vi "主动发送数据生成Condition(子VI).vi"(8 "数据发送协议":enum16{"2005-212协议", "2017-212协议"}(ring)=enum."2017-212协议", 9 "database":string, 10 "Label.Text":string, 11 "数值":i32) -> (3 "CONDITION":string)   [LabVIEW 2016, in "数据传输系统.lvlib"]
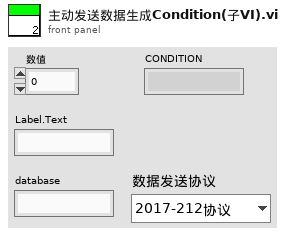
[diagram p1: front panel]
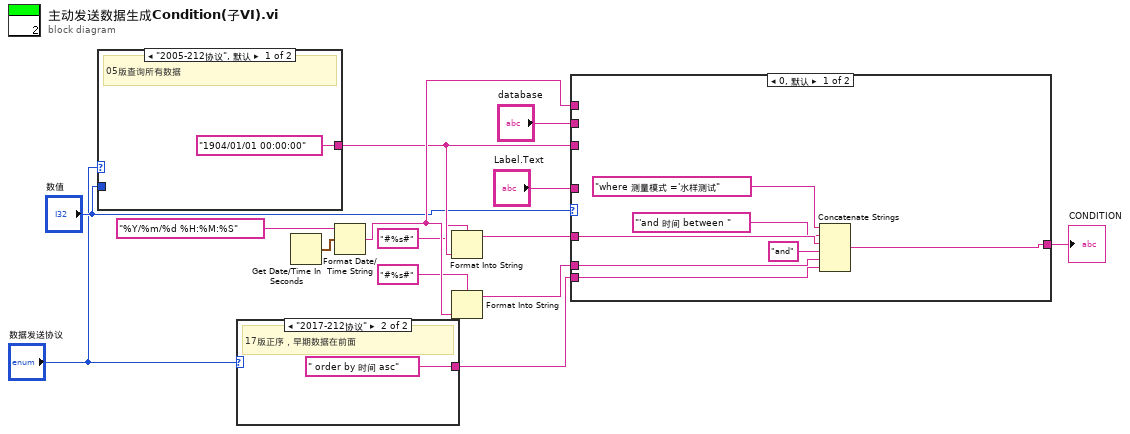
[diagram p0: block diagram]
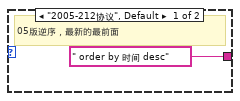
[diagram p2: hidden frame]
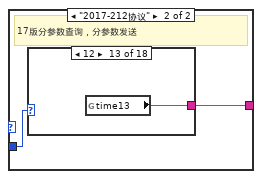
[diagram p3: hidden frame]
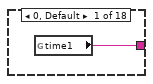
[diagram p4: hidden frame]
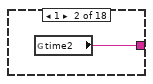
[diagram p5: hidden frame]
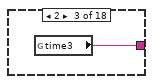
[diagram p6: hidden frame]
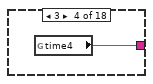
[diagram p7: hidden frame]
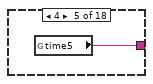
[diagram p8: hidden frame]
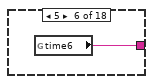
[diagram p9: hidden frame]
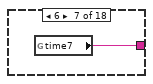
[diagram p10: hidden frame]
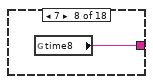
[diagram p11: hidden frame]
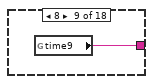
[diagram p12: hidden frame]
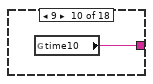
[diagram p13: hidden frame]
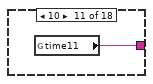
[diagram p14: hidden frame]
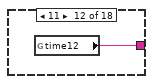
[diagram p15: hidden frame]
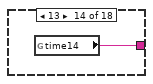
[diagram p16: hidden frame]
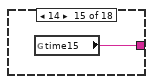
[diagram p17: hidden frame]
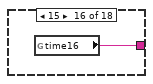
[diagram p18: hidden frame]
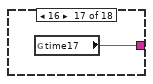
[diagram p19: hidden frame]
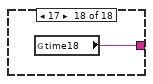
[diagram p20: hidden frame]
diagram:
  n1 = case shown="\"2005-212协议\", 默认" "数据发送协议" {
    tunnel: ["1904/01/01 00:00:00" w17] -> w13
    tunnel: "数值" -> [_ w16]
    frame "2005-212协议", Default {
      # "05版查询所有数据"
    }
    frame "2017-212协议" {
      # "17版分参数查询，分参数发送"
      n2 = case shown="12" w16 {
        tunnel: [w18 w19 w20 w21 w22 w23 w24 w25 w26 w27 w28 w29 w30 w31 w32 w33 w34 w35] -> w17
        frame 0, Default {
          n3 = global read "全局 水样时间.vi" "time1"() -> (w18:string)
        }
        frame 1 {
          n4 = global read "全局 水样时间.vi" "time2"() -> (w19:string)
        }
        frame 2 {
          n5 = global read "全局 水样时间.vi" "time3"() -> (w20:string)
        }
        frame 3 {
          n6 = global read "全局 水样时间.vi" "time4"() -> (w21:string)
        }
        frame 4 {
          n7 = global read "全局 水样时间.vi" "time5"() -> (w22:string)
        }
        frame 5 {
          n8 = global read "全局 水样时间.vi" "time6"() -> (w23:string)
        }
        frame 6 {
          n9 = global read "全局 水样时间.vi" "time7"() -> (w24:string)
        }
        frame 7 {
          n10 = global read "全局 水样时间.vi" "time8"() -> (w25:string)
        }
        frame 8 {
          n11 = global read "全局 水样时间.vi" "time9"() -> (w26:string)
        }
        frame 9 {
          n12 = global read "全局 水样时间.vi" "time10"() -> (w27:string)
        }
        frame 10 {
          n13 = global read "全局 水样时间.vi" "time11"() -> (w28:string)
        }
        frame 11 {
          n14 = global read "全局 水样时间.vi" "time12"() -> (w29:string)
        }
        frame 12 {
          n15 = global read "全局 水样时间.vi" "time13"() -> (w30:string)
        }
        frame 13 {
          n16 = global read "全局 水样时间.vi" "time14"() -> (w31:string)
        }
        frame 14 {
          n17 = global read "全局 水样时间.vi" "time15"() -> (w32:string)
        }
        frame 15 {
          n18 = global read "全局 水样时间.vi" "time16"() -> (w33:string)
        }
        frame 16 {
          n19 = global read "全局 水样时间.vi" "time17"() -> (w34:string)
        }
        frame 17 {
          n20 = global read "全局 水样时间.vi" "time18"() -> (w35:string)
        }
      }
    }
  }
  n21 = case shown="\"2017-212协议\"" "数据发送协议" {
    tunnel: [" order by 时间 desc" ("字符串") " order by 时间 asc" ("字符串")] -> w1
    frame "2005-212协议", Default {
      # "05版逆序，最新的最前面"
    }
    frame "2017-212协议" {
      # "17版正序，早期数据在前面"
    }
  }
  n22 = Get Date/Time In Seconds() -> (seconds since 1Jan1904=w5:timestamp)
  n23 = Format Date/Time String(time format string (%c)="%Y/%m/%d %H:%M:%S" ("时间格式字符串(%c)"), seconds (now)=w5) -> (date/time string=w14:string)  [unwired: 1 in]
  n24 = Format Into String(format string="#%s#" ("初始字符串"), w13) -> (resulting string=w7:string)  [unwired: 2 in, 1 out]
  n25 = Format Into String(format string="#%s#" ("初始字符串"), w14) -> (resulting string=w9:string)  [unwired: 2 in, 1 out]
  n26 = case shown="0, 默认" "数值" {
    selector: "数值" -> [_ w50]
    tunnel: w7 -> [w44 w55]
    tunnel: [w43 w56] -> w8
    tunnel: w9 -> [w41 w54]
    tunnel: "database" -> [_ w53]
    tunnel: "Label.Text" -> [_ w52]
    tunnel: w13 -> [_ w47]
    tunnel: w14 -> [_ w49]
    tunnel: w1 -> [w38 w45]
    frame 0, Default {
      n27 = Concatenate Strings("where 测量模式 ='水样测试" ("condition"), "'and 时间 between ", w44, "and" ("字符串"), w41, w38) -> (w43:string)
    }
    frame 14..17 {
      n28 = call "流量数据规范小时时间戳.vi"("字符串"=w47) -> ("result string"=w46:string)  [unwired: 10 in]
      n29 = call "database1查询.vi"("时间2"=w49, "table"=w52, "时间1"=w46, "database"=w53) -> ("error out"=w48:errorcluster, "data"=w51:string[][])  [unwired: 4 in, 1 out]
      n30 = call <vilib>:"Clear Errors.vi"("error in (no error)"=w48) -> ()  [unwired: 5 in, 2 out]
      n31 = Concatenate Strings(" where 时间 between ", w55, "and" ("字符串"), w54, w45) -> (w56:string)
      n32 = case shown="14" w50 {
        tunnel: w51 -> [_ w59 w60 w61 w62]
        frame 0, Default {
        }
        frame 14 {
          n33 = global write "全局流量数据小时.vi" "水位"(w59) -> ()
        }
        frame 15 {
          n34 = global write "全局流量数据小时.vi" "流速"(w60) -> ()
        }
        frame 16 {
          n35 = global write "全局流量数据小时.vi" "瞬时流量"(w61) -> ()
        }
        frame 17 {
          n36 = global write "全局流量数据小时.vi" "累积流量"(w62) -> ()
        }
      }
    }
  }
  "CONDITION" <- w8
